vi "PMX_GetMinValue.vi"(8 "Error in":errorcluster, 10 "Signal":refnum<k24>, 11 "Device":refnum<k24>) -> (0 "Error out":errorcluster, 2 "MinValue":dbl, 3 "Device":refnum<k24>)   [LabVIEW 2016]
doc: "Gets the minimum value of the given signal \n\nMaxValue: Minimum value of the given signal since last clear"
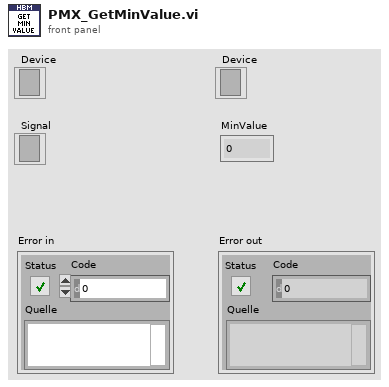
[diagram p1: front panel]
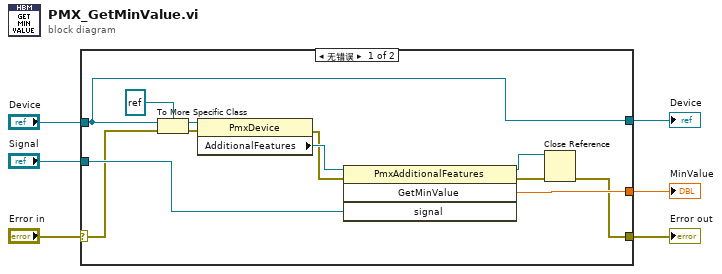
[diagram p0: block diagram]
diagram:
  n1 = case shown="无错误" "Error in" {
    selector: "Error in" -> [w11 w20]
    tunnel: [w7 w20] -> w4
    tunnel: "Device" -> [w14 w19]
    tunnel: [w14 w19] -> w5
    tunnel: "Signal" -> [w13 _]
    tunnel: [w12 _] -> w1
    frame No Error {
      n2 = To More Specific Class(target class=refnum<k24> refnum ("Zielklasse"), reference=w14, error in=w11) -> (specific class reference=w18:refnum<k24>, error out=w15:errorcluster)
      n3 = property on="Eigenschaftsknoten" class="PmxDevice"(reference=w18, error in=w15) -> (error out=w16:errorcluster, "AdditionalFeatures"=w17:refnum<k24>)  [unwired: 1 out]
      n4 = invoke on="Methodenknoten" class="PmxAdditionalFeatures" method="GetMinValue"(reference=w17, error in=w16, "signal"=w13) -> (reference out=w8:refnum<k24>, error out=w9:errorcluster, "GetMinValue"=w12:dbl)  [unwired: 1 in, 1 out]
      n5 = Close Reference(reference=w8, error in (no error)=w9) -> (error out=w7:errorcluster)
    }
    frame Error {
    }
  }
  "Device" <- w5
  "Error out" <- w4
  "MinValue" <- w1
